vi "ParseRequest.vi"(2 "Node html":string="index.html", 3 "String in":string="POST /index.htm HTTP/1.1\r\nHost: localhost:6263\r\nUser-Agent: Mozilla/5.0 (Macintosh; Intel Mac OS X 10_7_2) AppleWebKit/534.51.22 (KHTML, like Gecko) Version/5.1.1 Safari/534.51.22\r\nContent-Length: 11\r\nAccept: text/html,application/xhtml+xml,application/xml;q=0.9,*/*;q=0.8\r\nOrigin: http://localhost:6263\r\nContent-Type: application/x-www-form-urlencoded\r\nReferer: http://localhost:6263/index.htm\r\nAccept-Language: en-us\r\nAccept-Encoding: gzip, deflate\r\nConnection: keep-alive\r\n\r\n") -> (0 "Post size":i32, 1 "Reply":string="HTTP/1.1 200 OK\r\nUser-Agent: LabVIEW WebServer/0.1\nDate: Tue, 29 Nov 2011 19:10:36 GMT\nExpires: Tue, 29 Nov 2011 19:10:36 GMT\nIgnore-Buffer: xXxBUFFERxXx\nContent-Type: text/html\nContent-Length: 486\nConnection: keep-alive\r\n\r\n<!DOCTYPE HTML PUBLIC \"-//W3C//DTD HTML 4.0 Transitional//EN\">\n<HTML>\n<!-- Constructed with LabVIEW Report Generation -->\n<HEAD>\n<TITLE></TITLE>\n</HEAD>\n\n<BODY>\nthis is a test<!<IMG SRC=\"Tufts.png\" >>\n\n<form name=\"myform\" action=\"index.htm\" method=\"POST\">\n\n<br><br>\n<input type=\"submit\" name=\"fwd\" value=\"forward\"> \n<input type=\"submit\" name=\"1234\" value=\"left\"> \n<input type=\"submit\" name=\"12345\" value=\"back\"> \n<input type=\"submit\" name=\"12\" value=\"right\"> \n</form>\n\n</BODY>\n\n</HTML>\r\n\r\n")   [LabVIEW 2012]
doc: "Parses a message to or from a server"
panel:
  out "path 2":path=path "/Kim/Users/crogers/Desktop/TeleRobot/HTTPServer/docs/index.htm"
  out "array 2":string[](array[string])=["", "index.htm"]
  out "array":string[](array[string])
  in  "Error":string="<!DOCTYPE HTML PUBLIC \"-//W3C//DTD HTML 4.0 Transitional//EN\">\n<HTML>\n<HEAD>\n<TITLE>ERROR</TITLE>\n</HEAD>\n\n<BODY>\nSorry - no such webpage\n</BODY>\n</HTML>"
  out "path":path=path "/Kim/Users/crogers/Desktop/TeleRobot/HTTPServer/docs/index.htm"
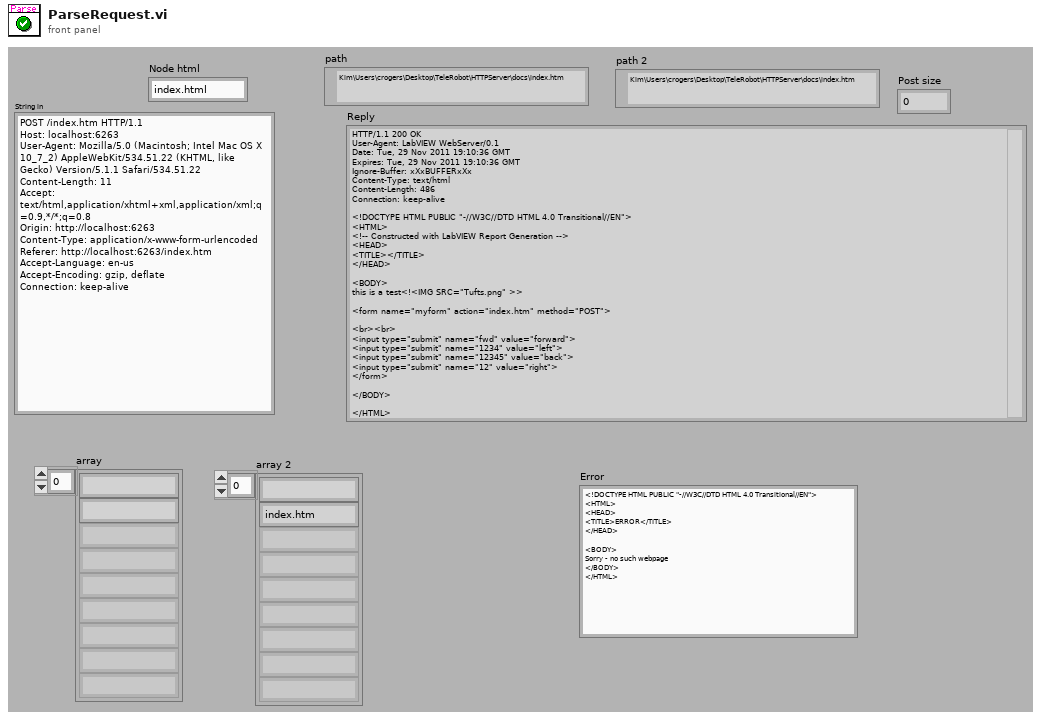
[diagram p1: front panel]
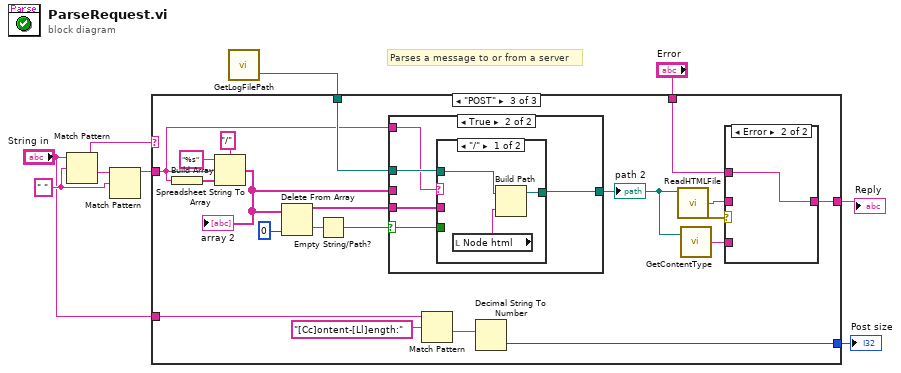
[diagram p0: block diagram]
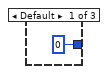
[diagram p2: hidden frame]
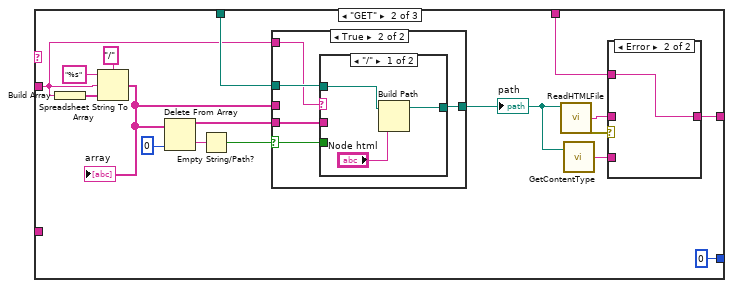
[diagram p3: hidden frame]
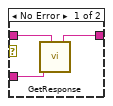
[diagram p4: hidden frame]
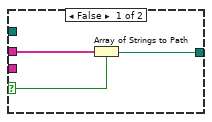
[diagram p5: hidden frame]
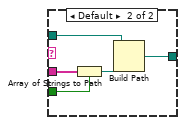
[diagram p6: hidden frame]
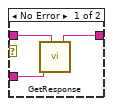
[diagram p7: hidden frame]
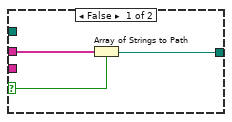
[diagram p8: hidden frame]
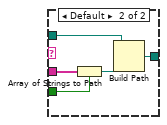
[diagram p9: hidden frame]
diagram:
  w7 = " " ("regular expression")
  # "Parses a message to or from a server"
  n1 = Match Pattern(string="String in", regular expression=w7) -> (before substring=w9:string, after substring=w8:string)  [unwired: 1 in, 2 out]
  n2 = Match Pattern(string=w8, regular expression=w7) -> (before substring=w6:string)  [unwired: 1 in, 3 out]
  n3 = call <userlib>:"GetLogFilePath.vi"() -> ("LogFolder"=w1:path)  [unwired: 2 in, 1 out]
  n4 = case shown="\"POST\"" w9 {
    tunnel: w6 -> [_ w13 w51]
    tunnel: w1 -> [_ w20 w60]
    tunnel: [_ w18 w58] -> w5
    tunnel: "Error" -> [_ w12 w53]
    tunnel: [0 0 w49] -> w3
    tunnel: "String in" -> [_ _ w48]
    frame Default {
    }
    frame "GET" {
      n5 = Build Array(w13) -> (w27:string[])
      n6 = Spreadsheet String To Array(delimiter (Tab)="/", format string="%s", spreadsheet string=w13, array type (2D Dbl)=w27) -> (array=w19:string[])
      "array" <- w19
      n7 = Delete From Array(array=w19, index=0) -> (deleted portion=w23:string, array with subset deleted=w21:string[])  [unwired: 1 in]
      n8 = Empty String/Path?(string/path=w23) -> (empty?=w22:bool)
      n9 = case shown="True" w22 {
        selector: w22 -> [w32 w39]
        tunnel: w21 -> [_ w38]
        tunnel: w20 -> [_ w37]
        tunnel: [w33 w36] -> w16
        tunnel: w19 -> [w34 _]
        tunnel: w13 -> [_ w35]
        frame False {
          n10 = Array of Strings to Path(0:w34, 1:w32) -> (2:w33:path)
        }
        frame True {
          n11 = case shown="\"/\"" w35 {
            tunnel: w39 -> [_ w47]
            tunnel: w38 -> [_ w46]
            tunnel: w37 -> [w42 w44]
            tunnel: [w41 w43] -> w36
            frame "/" {
              n12 = Build Path(base path=w42, name or relative path="Node html") -> (appended path=w41:path)
            }
            frame Default {
              n13 = Array of Strings to Path(0:w46, 1:w47) -> (2:w45:path)
              n14 = Build Path(base path=w44, name or relative path=w45) -> (appended path=w43:path)
            }
          }
        }
      }
      "path" <- w16
      n15 = call <userlib>:"ReadHTMLFile.vi"("file path (dialog if empty)"=w16) -> ("contents"=w15:string, "error out"=w14:errorcluster)  [unwired: 6 in, 1 out]
      n16 = call <userlib>:"GetContentType.vi"("File Path"=w16) -> ("Content Type"=w17:string)  [unwired: 1 in]
      n17 = case shown="Error" w14 {
        tunnel: [w28 w31] -> w18
        tunnel: w15 -> [w29 _]
        tunnel: w17 -> [w30 _]
        tunnel: w12 -> [_ w31]
        frame No Error {
          n18 = call <userlib>:"GetResponse.vi"("Content Type"=w30, "ResponseBody"=w29) -> ("TotalResponseOut"=w28:string)  [unwired: 3 in]
        }
        frame Error {
        }
      }
    }
    frame "POST" {
      n19 = Build Array(w51) -> (w67:string[])
      n20 = Spreadsheet String To Array(delimiter (Tab)="/", format string="%s", spreadsheet string=w51, array type (2D Dbl)=w67) -> (array=w59:string[])
      "array 2" <- w59
      n21 = Delete From Array(array=w59, index=0) -> (deleted portion=w63:string, array with subset deleted=w61:string[])  [unwired: 1 in]
      n22 = Empty String/Path?(string/path=w63) -> (empty?=w62:bool)
      n23 = case shown="True" w62 {
        selector: w62 -> [w72 w79]
        tunnel: w61 -> [_ w78]
        tunnel: w60 -> [_ w77]
        tunnel: [w73 w76] -> w56
        tunnel: w59 -> [w74 _]
        tunnel: w51 -> [_ w75]
        frame False {
          n24 = Array of Strings to Path(0:w74, 1:w72) -> (2:w73:path)
        }
        frame True {
          n25 = case shown="\"/\"" w75 {
            tunnel: w79 -> [_ w87]
            tunnel: w78 -> [_ w86]
            tunnel: w77 -> [w82 w84]
            tunnel: [w81 w83] -> w76
            frame "/" {
              n26 = local read "Node html"() -> (w80:string)
              n27 = Build Path(base path=w82, name or relative path=w80) -> (appended path=w81:path)
            }
            frame Default {
              n28 = Array of Strings to Path(0:w86, 1:w87) -> (2:w85:path)
              n29 = Build Path(base path=w84, name or relative path=w85) -> (appended path=w83:path)
            }
          }
        }
      }
      "path 2" <- w56
      n30 = Match Pattern(string=w48, regular expression="[Cc]ontent-[Ll]ength:" ("match string")) -> (after substring=w50:string)  [unwired: 1 in, 3 out]
      n31 = Decimal String To Number(string=w50) -> (number=w49:i32)  [unwired: 3 out]
      n32 = call <userlib>:"ReadHTMLFile.vi"("file path (dialog if empty)"=w56) -> ("contents"=w55:string, "error out"=w54:errorcluster)  [unwired: 6 in, 1 out]
      n33 = call <userlib>:"GetContentType.vi"("File Path"=w56) -> ("Content Type"=w57:string)  [unwired: 1 in]
      n34 = case shown="Error" w54 {
        tunnel: [w68 w71] -> w58
        tunnel: w55 -> [w69 _]
        tunnel: w57 -> [w70 _]
        tunnel: w53 -> [_ w71]
        frame No Error {
          n35 = call <userlib>:"GetResponse.vi"("Content Type"=w70, "ResponseBody"=w69) -> ("TotalResponseOut"=w68:string)  [unwired: 3 in]
        }
        frame Error {
        }
      }
    }
  }
  "Reply" <- w5
  "Post size" <- w3
